vi "Device name set.vi"(8 "error in":errorcluster, 9 "Channel list":tag[][](array[tag]), 10 "Message":string, 11 "Module ID":i32=-1) -> (0 "error out":errorcluster)   [LabVIEW 2025, in "NI DAQ Aug 25.lvlib"]
doc: "Triggers after the name of the device has been changed.\n\n_____\nCreated using DQMH Framework: Event Scripter 7.1.1.1528."
uses:
  NI DAQ Aug 25.lvlib
  Device name set Argument--cluster.ctl
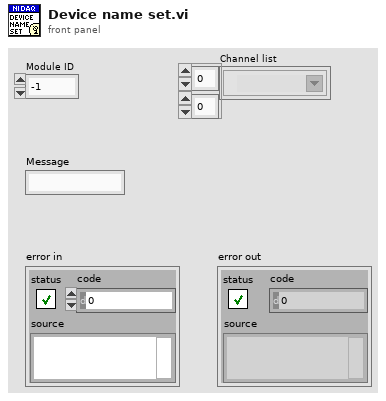
[diagram p1: front panel]
types:
  T1 = typedef "NI DAQ Aug 25.lvlib/Device name set Argument--cluster.ctl" = cluster{"Module ID":i32, "Message":string, "Channel list":tag[][]}
  T2 = typedef "NI DAQ Aug 25.lvlib/Broadcast Events--cluster.ctl" = cluster{"Module Did Init":refnum<user-event>, "Status Updated":refnum<user-event>, "Error Reported":refnum<user-event>, "Module Did Stop":refnum<user-event>, "Update Module Execution Status":refnum<user-event>, "Device name set":refnum<user-event>}
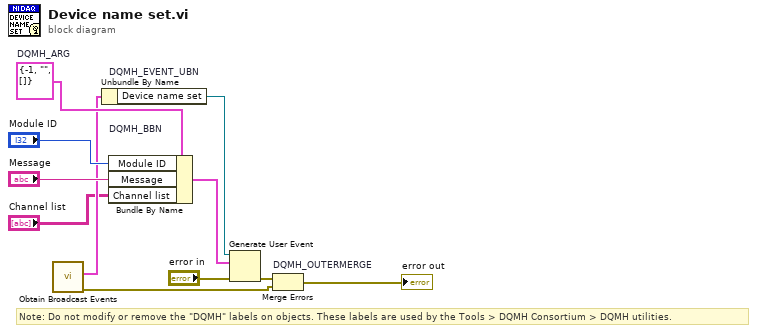
[diagram p0: block diagram]
diagram:
  w6 = T1 {"Module ID"=-1, "Message"="", "Channel list"=[]}  # DQMH_ARG
  # "Note: Do not modify or remove the \"DQMH\" labels on objects. These labels are used by the Tools > DQMH Consortium > DQMH utilities."
  n1 = call "Obtain Broadcast Events.vi"() -> ("error out"=w3:errorcluster, "NI DAQ Aug 25 Broadcast Events"=w2:T2)  [unwired: 10 in]
  n2 = Unbundle By Name "DQMH_EVENT_UBN"(w2) -> ("Device name set"=w8:refnum<user-event>)
  n3 = Bundle By Name "DQMH_BBN"(cluster=w6, "Module ID"="Module ID", "Message"="Message", "Channel list"="Channel list") -> (w9:T1)
  n4 = Generate User Event(user event=w8, event data cluster=w9, error in="error in") -> (error out=w7:errorcluster)  [unwired: 1 in, 1 out]
  n5 = Merge Errors "DQMH_OUTERMERGE"(w7, w3) -> (→"error out":errorcluster)
